vi "brc_daq_stop_DAQ.vi"(5 "error in (no error)":errorcluster, 6 "mHandle":i32) -> (19 "error out":errorcluster)   [LabVIEW 2019, in "BRC-DAQ.lvlib"]
uses:
  BRC-DAQ.lvlib
panel:
  out "return_value":i32
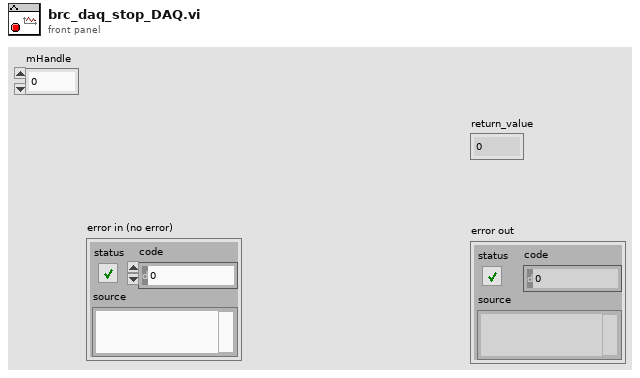
[diagram p1: front panel]
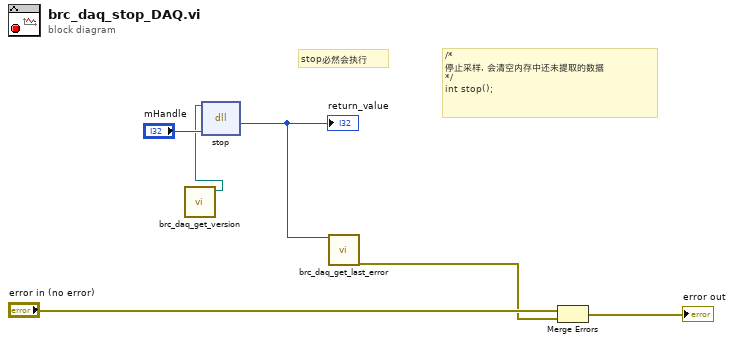
[diagram p0: block diagram]
diagram:
  # "/*\n停止采样, 会清空内存中还未提取的数据\n*/\nint stop();"
  # "stop必然会执行"
  n1 = call "brc_daq_get_version.vi"() -> ("dll path"=w1:path)  [unwired: 11 in]
  n2 = dll-call lib="E:/01 BRC project/04BRC-daq/04 Drive/DAQ-x64/DLL/brc_daq_sdk.dll" fn="stop"(path in=w1, "mHandle"="mHandle") -> ("return type"=w4:i32)  [unwired: 3 in, 2 out]
  "return_value" <- w4
  n3 = call "brc_daq_get_last_error.vi"("return_value"=w4) -> ("error out"=w3:errorcluster)  [unwired: 18 in]
  n4 = Merge Errors("error in (no error)", w3) -> (→"error out":errorcluster)
